vi "Angle_Motor_Pid.vi"(11 "MotorControlDevRef":T1) -> ()   [LabVIEW 2020]
uses:
  <vilib>/Rock Robotics/WPI/MotorControl/WPI_MotorControlDeviceRef.ctl
  <vilib>/Rock Robotics/WPI/MotorControl/WPI_MotorControlType.ctl
  <vilib>/Rock Robotics/SystemInterfaces/DIO/FPGA_DIOPWMChannel.ctl
  <vilib>/Rock Robotics/WPI/PWM/WPI_PWMDeadband.ctl
  <vilib>/Rock Robotics/SystemInterfaces/DIO/FPGA_DIOChannel.ctl
  Robot Global Data.vi
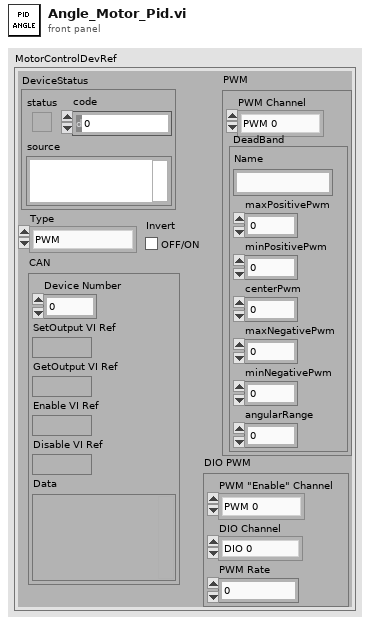
[diagram p1: front panel]
types:
  T1 = typedef "WPI_MotorControlDeviceRef.ctl" = cluster{"DeviceStatus":errorcluster, "Type":T2, "PWM":cluster{"PWM Channel":T3, "DeadBand":T4}, "CAN":cluster{"Device Number":u8, "SetOutput VI Ref":variant, "GetOutput VI Ref":variant, "Enable VI Ref":variant, "Disable VI Ref":variant, "Data":variant}, "Invert":bool, "DIO PWM":cluster{"PWM \"Enable\" Channel":T3, "DIOChannel":T5, "PWM Rate":dbl}}
  T2 = typedef "WPI_MotorControlType.ctl" = enum16{"PWM", "CAN", "DIO PWM"}
  T3 = typedef "FPGA_DIOPWMChannel.ctl" = enum8{"PWM 0", "PWM 1", "PWM 2", "PWM 3", "PWM 4", "PWM 5", "PWM 6", "PWM 7", "PWM 8", "PWM 9", "PWM MXP 0", "PWM MXP 1", "PWM MXP 2", "PWM MXP 3", "PWM MXP 4", "PWM MXP 5", "PWM MXP 6", "PWM MXP 7", "PWM MXP 8", "PWM MXP 9", "Invalid"}
  T4 = typedef "WPI_PWMDeadband.ctl" = cluster{"Name":string, "maxPositivePwm":i32, "minPositivePwm":i32, "centerPwm":i32, "maxNegativePwm":i32, "minNegativePwm":i32, "angularRange":u16}
  T5 = typedef "FPGA_DIOChannel.ctl" = enum8{"DIO 0", "DIO 1", "DIO 2", "DIO 3", "DIO 4", "DIO 5", "DIO 6", "DIO 7", "DIO 8", "DIO 9", "DIO MXP 0", "DIO MXP 1", "DIO MXP 2", "DIO MXP 3", "DIO MXP 4", "DIO MXP 5", "DIO MXP 6", "DIO MXP 7", "DIO MXP 8", "DIO MXP 9", "DIO MXP 10", "DIO MXP 11", "DIO MXP 12", "DIO MXP 13", "DIO MXP 14", "DIO MXP 15", "SPI Port CS1", "SPI Port CS2", "SPI Port CS3", "SPI Port MISO", "SPI Port MOSI", "Invalid"}
  T6 = typedef "Trajectory_Library.lvlib/SWERVE_DRIVE_MODULE_STATE.ctl" = cluster{"Speed":dbl, "Angle":T7}
  T7 = typedef "Trajectory_Library.lvlib/ROTATION2D.ctl" = cluster{"VALUE":dbl, "COS":dbl, "SIN":dbl}
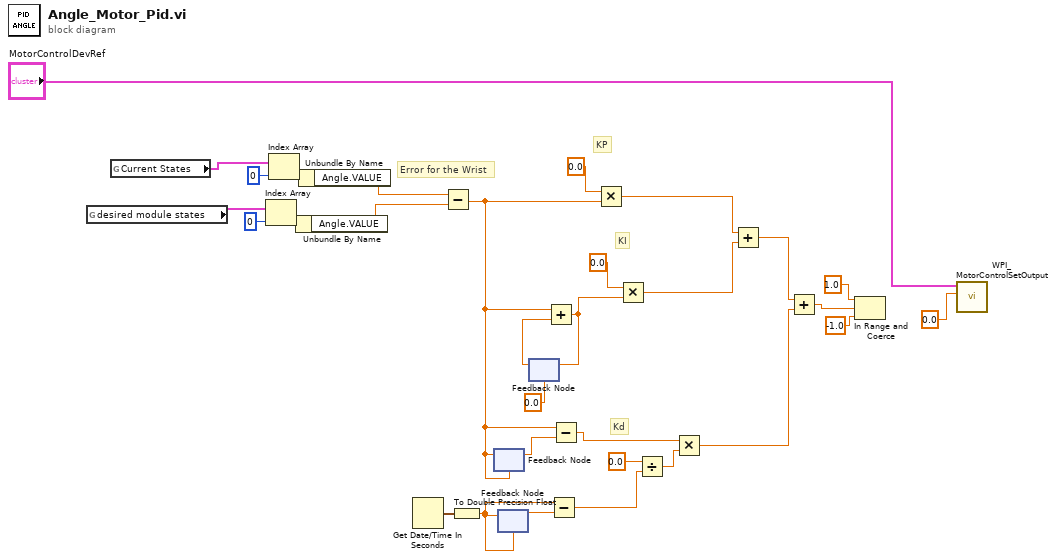
[diagram p0: block diagram]
diagram:
  # "Kd"
  # "KI"
  # "Error for the Wrist"
  # "KP"
  n1 = global read "Robot Global Data.vi" "desired module states"() -> (w3:T6[])
  n2 = global read "Robot Global Data.vi" "Current States"() -> (w9:T6[])
  n3 = Index Array(array=w3, index=0) -> (element=w4:T6)
  n4 = Index Array(array=w9, index=0) -> (element=w8:T6)
  n5 = Unbundle By Name(w4) -> ("Angle.VALUE"=w2:dbl)
  n6 = Unbundle By Name(w8) -> ("Angle.VALUE"=w6:dbl)
  n7 = Get Date/Time In Seconds() -> (seconds since 1Jan1904=w25:timestamp)
  n8 = Subtract(x=w6, y=w2) -> (x-y=w10:dbl)
  n9 = To Double Precision Float(number=w25) -> (double precision float=w23:dbl)
  n10 = feedback #1(w10) -> (w15:dbl)
  n11 = feedback-in #1(w10) -> ()
  n12 = feedback #2(w23) -> (w24:dbl)
  n13 = feedback-in #2(w23) -> ()
  n14 = feedback #3(0.0) -> (w29:dbl)
  n15 = Add(x=w10, y=w29) -> (x+y=w26:dbl)
  n16 = feedback-in #3(w26) -> ()
  n17 = Subtract(x=w23, y=w24) -> (x-y=w14:dbl)
  n18 = Subtract(x=w10, y=w15) -> (x-y=w16:dbl)
  n19 = Multiply(x=0.0 ("y"), y=w10) -> (x*y=w18:dbl)
  n20 = Multiply(x=0.0 ("y"), y=w26) -> (x*y=w21:dbl)
  n21 = Divide(x=0.0, y=w14) -> (x/y=w13:dbl)
  n22 = Multiply(x=w16, y=w13) -> (x*y=w20:dbl)
  n23 = Add(x=w18, y=w21) -> (x+y=w17:dbl)
  n24 = Add(x=w17, y=w20) -> (x+y=w12:dbl)
  n25 = In Range and Coerce(upper limit=1.0, x=w12, lower limit=-1.0) -> ()  [unwired: 2 out]
  n26 = call <vilib>:"WPI_MotorControlSetOutput.vi"("Output"=0.0, "MotorControlDevRef"="MotorControlDevRef") -> ()  [unwired: 7 in, 3 out]
